vi "Ping Network.vi"(8 "error in (no error)":errorcluster, 11 "Network Test in":refnum<class "Network Test.lvclass">) -> (0 "error out":errorcluster, 1 "Response":string, 2 "PingSuccess?":bool, 3 "Network Test out":refnum<class "Network Test.lvclass">)   [LabVIEW 2017, in "Network Test.lvlib" / "Network Test.lvclass"]
uses:
  Network Test.lvclass
  Network Test.lvclass/Network Test.ctl
panel:
  out "Status":i32(ring) items=["Success"=0, "DestinationNetworkUnreachable"=11002, "DestinationHostUnreachable"=11003, "DestinationProhibited, DestinationProtocolUnreachable"=11004, "DestinationPortUnreachable"=11005, "NoResources"=11006, "BadOption"=11007, "HardwareError"=11008, "PacketTooBig"=11009, "TimedOut"=11010, "BadRoute"=11012, "TtlExpired"=11013, "TtlReassemblyTimeExceeded"=11014, "ParameterProblem"=11015, "SourceQuench"=11016, "BadDestination"=11018, "DestinationUnreachable"=11040, "TimeExceeded"=11041, "BadHeader"=11042, "UnrecognizedNextHeader"=11043, "IcmpError"=11044, "DestinationScopeMismatch"=11045, "Unknown"=-1]
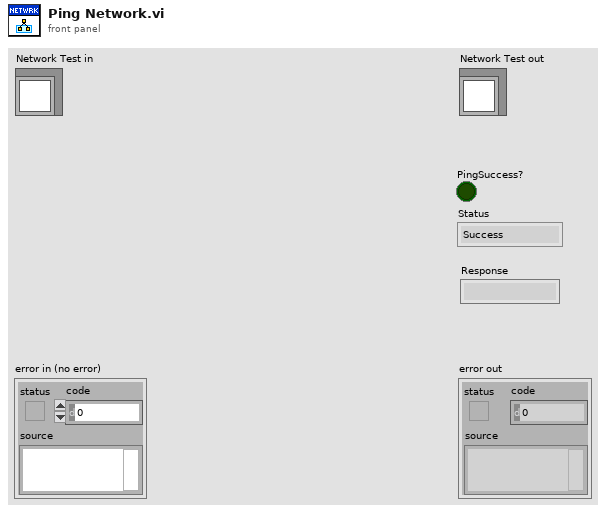
[diagram p1: front panel]
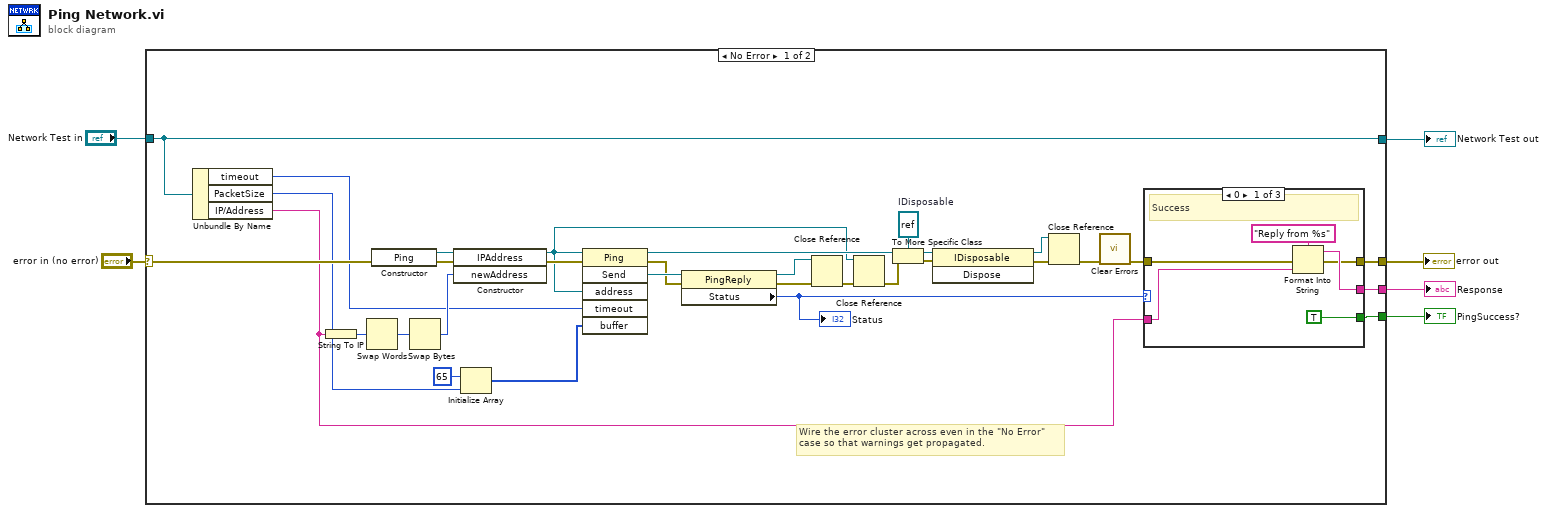
[diagram p0: block diagram]
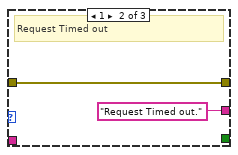
[diagram p2: hidden frame]
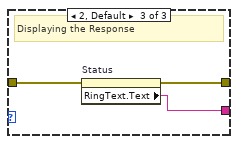
[diagram p3: hidden frame]
diagram:
  # "Wire the error cluster across even in the \"No Error\"\ncase so that warnings get propagated."
  n1 = case shown="No Error" "error in (no error)" {
    selector: "error in (no error)" -> [w11 w51]
    tunnel: [w15 _] -> w3
    tunnel: [w14 _] -> w4
    tunnel: [w12 w51] -> w1
    tunnel: "Network Test in" -> [w7 w50]
    tunnel: [w7 w50] -> w2
    frame No Error {
      w29 = refnum<k24> refnum  # IDisposable
      n2 = Unbundle By Name(w7) -> ("timeout"=w8:i32, "PacketSize"=w9:i32, "IP/Address"=w10:string)
      n3 = String To IP(1:w10) -> (0:w33:u32)
      n4 = Swap Words(1:w33) -> (0:w31:u32)
      n5 = constructor class="Ping"(error in=w11) -> (reference out=w38:refnum<k24>, error out=w35:errorcluster)  [unwired: 2 in, 1 out]
      n6 = Swap Bytes(anything=w31) -> (byte swapped=w32:u32)
      n7 = constructor class="IPAddress"(error in=w35, "newAddress"=w32) -> (reference out=w25:refnum<k24>, error out=w34:errorcluster)  [unwired: 2 in, 2 out]
      n8 = Initialize Array(65, w9) -> (w37:i32[])
      n9 = invoke class="Ping" method="Send"(reference=w38, error in=w34, "address"=w25, "timeout"=w8, "buffer"=w37) -> (reference out=w30:refnum<k24>, error out=w17:errorcluster, "Send"=w18:refnum<k24>)  [unwired: 1 in, 3 out]
      n10 = property class="PingReply"(reference=w18, error in=w17) -> (reference out=w28:refnum<k24>, error out=w27:errorcluster, "Status"=w16:i32)
      "Status" <- w16
      n11 = Close Reference(reference=w28, error in (no error)=w27) -> (error out=w26:errorcluster)
      n12 = Close Reference(reference=w25, error in (no error)=w26) -> (error out=w24:errorcluster)
      n13 = To More Specific Class(target class=w29, reference=w30, error in=w24) -> (specific class reference=w23:refnum<k24>, error out=w22:errorcluster)
      n14 = invoke class="IDisposable" method="Dispose"(reference=w23, error in=w22) -> (reference out=w20:refnum<k24>, error out=w21:errorcluster)  [unwired: 1 in, 1 out]
      n15 = Close Reference(reference=w20, error in (no error)=w21) -> (error out=w19:errorcluster)
      n16 = call <vilib>:"Clear Errors.vi"("error in (no error)"=w19) -> ("error out"=w13:errorcluster)  [unwired: 5 in, 1 out]
      n17 = case shown="0" w16 {
        tunnel: w10 -> [w44 _ _]
        tunnel: [w43 "Request Timed out." w47] -> w15
        tunnel: [TRUE _ _] -> w14
        tunnel: w13 -> [w41 w45 w49]
        tunnel: [w40 w45 w48] -> w12
        frame 0 {
          # "Success"
          n18 = Format Into String(format string="Reply from %s", error in=w41, w44) -> (resulting string=w43:string, error out=w40:errorcluster)  [unwired: 1 in]
        }
        frame 1 {
          # "Request Timed out"
        }
        frame 2, Default {
          # "Displaying the Response"
          n19 = property on="Status" class="Ring (strict)"(error in=w49) -> (error out=w48:errorcluster, "RingText.Text"=w47:string)  [unwired: 1 in, 1 out]
        }
      }
    }
    frame Error {
    }
  }
  "error out" <- w1
  "Network Test out" <- w2
  "Response" <- w3
  "PingSuccess?" <- w4
